vi "Get Driver Alias Array.vi"(8 "error in (no error)":errorcluster, 11 "Instrument Handler in":refnum<class "Instrument Handler.lvclass">) -> (0 "error out":errorcluster, 2 "Driver Alias Array":T1[](array[typedef]), 3 "Instrument Handler out":refnum<class "Instrument Handler.lvclass">)   [LabVIEW 2020, in "Instrument Handler.lvlib" / "Instrument Handler.lvclass"]
doc: "List the Driver Alias arrays contained in the Alias table."
uses:
  Instrument Handler.lvclass
  Controls/Ctl_DriverAliasElement.ctl
  Instrument Handler.lvclass/Instrument Handler.ctl
  Instrument Handler.lvlib
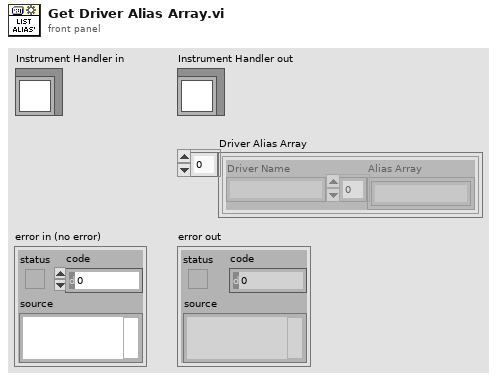
[diagram p1: front panel]
types:
  T1 = typedef "Instrument Handler.lvlib/Ctl_DriverAliasElement.ctl" = cluster{"Driver Name":string, "Alias Array":string[]}
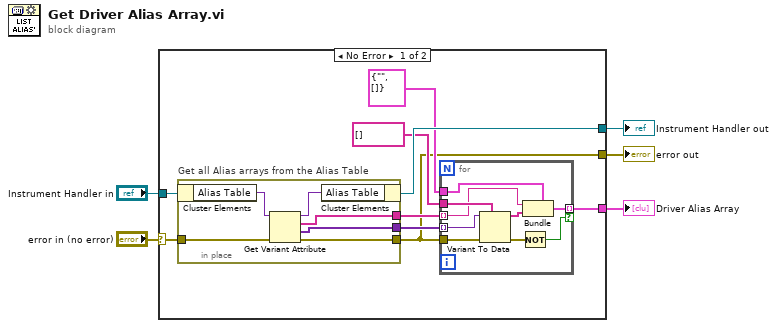
[diagram p0: block diagram]
diagram:
  n1 = case shown="No Error" "error in (no error)" {
    selector: "error in (no error)" -> [w12 w31]
    tunnel: [w7 w31] -> w4
    tunnel: [w13 w30] -> w2
    tunnel: "Instrument Handler in" -> [w14 w30]
    tunnel: [w6 _] -> w1
    frame No Error {
      n2 = in-place "Get all Alias arrays from the Alias Table" {
        in-place-border: w12 -> [w27]
        in-place-border: [w26] -> w7
        in-place-border: [w25] -> w11
        in-place-border: [w24] -> w10
        n3 = in-place-cluster #1(w14) -> ("Alias Table"=w29:variant)
        n4 = Get Variant Attribute(Variant=w29, error in=w27) -> (duplicate Variant=w28:variant, names=w24:string[], values=w25:variant[], error out=w26:errorcluster)  [unwired: 2 in]
        n5 = in-place-cluster #1("Alias Table"=w28) -> (w13:refnum<class "Instrument Handler.lvclass">)
      }
      n6 = for {
        tunnel: w11 -> [w23] mode=indexing
        tunnel: w7 -> [w22]
        tunnel: w10 -> [w19] mode=indexing
        tunnel: string[] [] -> [w21]
        tunnel: T1 {"Driver Name"="", "Alias Array"=[]} -> [w20]
        tunnel: [w17] -> w6 mode=indexing if=w15
        n7 = Variant To Data(error in=w22, type=w21, Variant=w23) -> (data=w18:string[], error out=w16:errorcluster)
        n8 = Not(x=w16) -> (.not. x?=w15:bool)
        n9 = Bundle(cluster=w20, "Driver Name"=w19, "Alias Array"=w18) -> (w17:T1)
      }
    }
    frame Error {
    }
  }
  "error out" <- w4
  "Instrument Handler out" <- w2
  "Driver Alias Array" <- w1
